vi "Pop.vi"(3 "Error In":errorcluster, 4 "Delete?":bool, 5 "object in":refnum<class "Stack.lvclass">) -> (0 "Error Out":errorcluster, 1 "Data":variant, 2 "object out":refnum<class "Stack.lvclass">)   [LabVIEW 2024, in "Stack.lvclass"]
uses:
  Stack.lvclass
  Stack.lvclass/Stack.ctl
panel:
  # "Connector Pane"
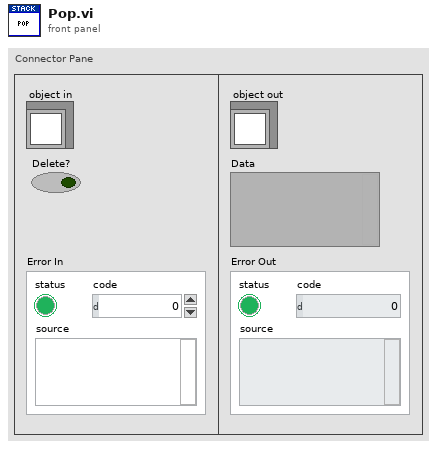
[diagram p1: front panel]
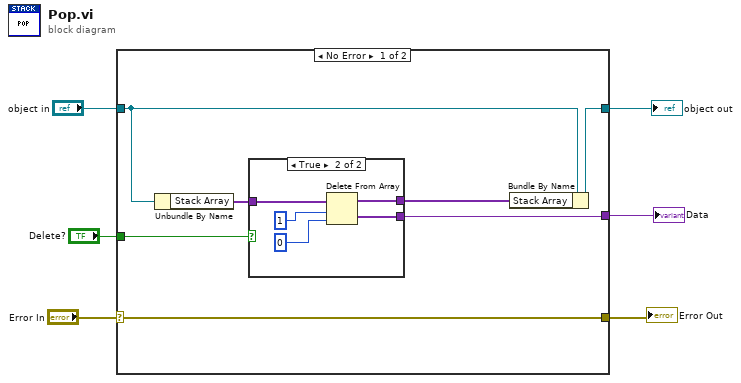
[diagram p0: block diagram]
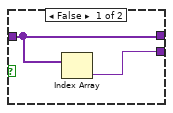
[diagram p2: hidden frame]
diagram:
  n1 = case shown="No Error" "Error In" {
    selector: "Error In" -> [w13 w22]
    tunnel: [w13 w22] -> w5
    tunnel: [w10 w21] -> w3
    tunnel: "object in" -> [w12 w21]
    tunnel: [w8 _] -> w2
    tunnel: "Delete?" -> [w7 _]
    frame No Error {
      n2 = Unbundle By Name(w12) -> ("Stack Array"=w11:variant[])
      n3 = case shown="True" w7 {
        tunnel: w11 -> [w14 w20]
        tunnel: [w14 w18] -> w9
        tunnel: [w15 w16] -> w8
        frame False {
          n4 = Index Array(array=w14) -> (element=w15:variant)  [unwired: 1 in]
        }
        frame True {
          n5 = Delete From Array(array=w20, length=1, index=0) -> (deleted portion=w16:variant[], array with subset deleted=w18:variant[])
        }
      }
      n6 = Bundle By Name(cluster=w12, "Stack Array"=w9) -> (w10:refnum<class "Stack.lvclass">)
    }
    frame Error {
    }
  }
  "Error Out" <- w5
  "object out" <- w3
  "Data" <- w2
